vi "CRYRead format string.vi"(11 "Format string":string) -> (0 "Notation":u16(slide), 1 "Digits":u16, 2 "Precision":u16(ring) items=["Digits of precision", "Significant digits"], 3 "Hide Traling Zeros":bool)   [LabVIEW 2013]
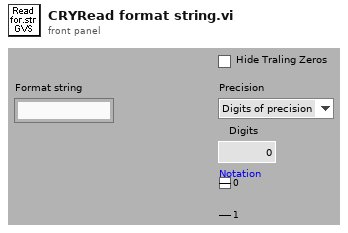
[diagram p1: front panel]
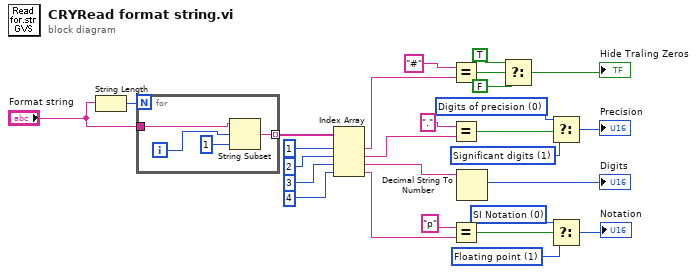
[diagram p0: block diagram]
diagram:
  w9 = u16 1 items=["SI Notation", "Floating point"] ("Notation")
  w10 = u16 0 items=["SI Notation", "Floating point"] ("Notation")
  w14 = u16 0 items=["Digits of precision", "Significant digits"] ("Precision")
  w13 = u16 1 items=["Digits of precision", "Significant digits"] ("Precision")
  n1 = String Length(string="Format string") -> (length=w26:i32)
  n2 = for {
    N: w26 -> [_]
    tunnel: "Format string" -> [w30]
    tunnel: [w28] -> w25 mode=indexing
    i -> [w29]
    n3 = String Subset(string=w30, offset (0)=w29, length (rest)=1 ("length (rest)")) -> (substring=w28:string)
  }
  n4 = Index Array(array=w25, index #1=1 ("index"), index #2=2 ("index"), index #3=3 ("index"), index #4=4 ("index")) -> (element #1=w8:string, element #2=w7:string, element #3=w6:string, element #4=w5:string)
  n5 = Equal?(x="#" ("format string"), y=w8) -> (x = y?=w19:bool)
  n6 = Equal?(x="." ("format string"), y=w7) -> (x = y?=w15:bool)
  n7 = Equal?(x="p" ("format string"), y=w5) -> (x = y?=w11:bool)
  n8 = Decimal String To Number(string=w6) -> (number=→"Digits":i32)  [unwired: 2 in, 1 out]
  n9 = Select(t=TRUE ("Revert"), s=w19, f=FALSE) -> (s? t:f=→"Hide Traling Zeros":bool)
  n10 = Select(t=w14, s=w15, f=w13) -> (s? t:f=→"Precision":u16)
  n11 = Select(t=w10, s=w11, f=w9) -> (s? t:f=→"Notation":u16)
